vi "Create Test Pattern.vi"() -> ()   [LabVIEW 2016]
panel:
  in  "File Path Control":path
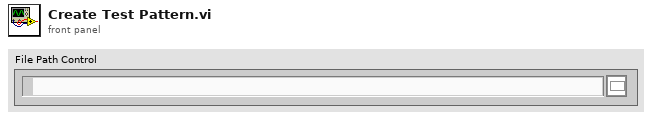
[diagram p1: front panel]
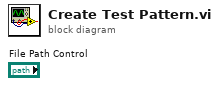
[diagram p0: block diagram]
diagram:
